vi "New From Listener.vi"(4 "Immutable TLS":refnum<k36>, 6 "TLS":bool, 7 "From":refnum<class "Endpoint.lvclass">, 10 "TCP Connection":refnum<k5>, 11 "URI":refnum<class "URI.lvclass">) -> (0 "error out":errorcluster, 3 "Client":refnum<class "Websocket Client.lvclass">)   [LabVIEW 2020, in "Stream-Websocket.lvlib" / "Websocket Client.lvclass"]
uses:
  Websocket Client.lvclass
  <vilib>/IlluminatedG/lv-stream/URI/URI.lvclass
  <vilib>/IlluminatedG/lv-stream/Endpoint/Endpoint.lvclass
  C:/Program Files (x86)/National Instruments/LabVIEW 2020/vi.lib/IlluminatedG/lv-stream/Endpoint/Endpoint.lvclass
  C:/Program Files (x86)/National Instruments/LabVIEW 2020/vi.lib/IlluminatedG/lv-stream/Connection/Connection.lvclass
  Websocket Client.lvclass/Websocket Client.ctl
  <vilib>/IlluminatedG/lv-stream/Connection State.ctl
  <vilib>/IlluminatedG/lv-stream/Connection/State.ctl
  <vilib>/IlluminatedG/lv-stream/Stream.lvlib
  <vilib>/IlluminatedG/lv-stream/Connection/Connection.lvclass
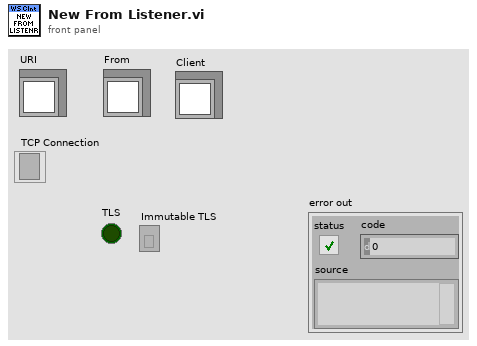
[diagram p1: front panel]
types:
  T1 = typedef "Stream.lvlib/Connection.lvclass/State.ctl" = enum16{"Closed", "Idle", "Connecting", "Connected", "Shutdown"}
  T2 = typedef "Stream.lvlib/Connection State.ctl" = enum16{"Connected", "Disconnected"}
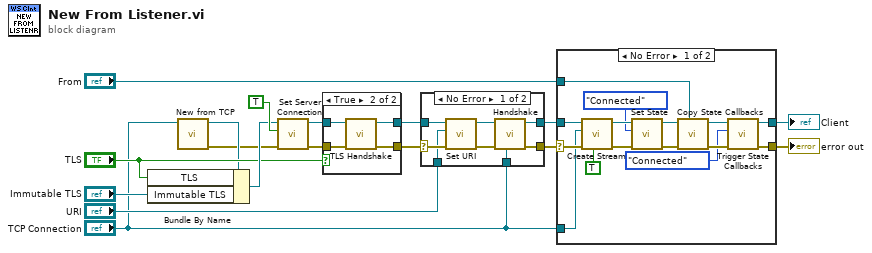
[diagram p0: block diagram]
diagram:
  n1 = call "New from TCP.vi"("TCP Connection"="TCP Connection") -> ("error out"=w2:errorcluster, "Websocket Client out"=w3:refnum<class "Websocket Client.lvclass">)  [unwired: 9 in]
  n2 = Bundle By Name(cluster=w3, "TLS"="TLS", "Immutable TLS"="Immutable TLS") -> (w9:refnum<class "Websocket Client.lvclass">)
  n3 = call "Set Server Connection.vi"("error in (no error)"=w2, "Server Connection"=TRUE, "Websocket Client in"=w9) -> ("error out"=w7:errorcluster, "Websocket Client out"=w8:refnum<class "Websocket Client.lvclass">)  [unwired: 7 in]
  n4 = case shown="True" "TLS" {
    tunnel: w8 -> [w18 w23]
    tunnel: w7 -> [w19 w22]
    tunnel: [w19 w21] -> w6
    tunnel: [w18 w20] -> w5
    frame False {
    }
    frame True {
      n5 = call "TLS Handshake.vi"("error in (no error)"=w22, "Websocket Client in"=w23) -> ("error out"=w21:errorcluster, "Websocket Client out"=w20:refnum<class "Websocket Client.lvclass">)  [unwired: 8 in]
    }
  }
  n6 = case shown="No Error" w6 {
    selector: w6 -> [w31 w33]
    tunnel: "URI" -> [w30 _]
    tunnel: [w27 w33] -> w13
    tunnel: [w26 w32] -> w12
    tunnel: "TCP Connection" -> [w25 _]
    tunnel: w5 -> [w24 w32]
    frame No Error {
      n7 = call <vilib>:"Set URI.vi"("error in (no error)"=w31, "URI"=w30, "Endpoint in"=w24) -> ("error out"=w28:errorcluster, "Endpoint out"=w29:refnum<class "Websocket Client.lvclass">)  [unwired: 7 in]
      n8 = call "Handshake.vi"("TCP Connection"=w25, "error in (no error)"=w28, "Websocket Client in"=w29) -> ("error out"=w27:errorcluster, "Websocket Client out"=w26:refnum<class "Websocket Client.lvclass">)  [unwired: 7 in]
    }
    frame Error {
    }
  }
  n9 = case shown="No Error" w13 {
    selector: w13 -> [w47 w49]
    tunnel: w12 -> [w48 w50]
    tunnel: "TCP Connection" -> [w46 _]
    tunnel: "From" -> [w38 _]
    tunnel: [w37 w50] -> w15
    tunnel: [w36 w49] -> w14
    frame No Error {
      n10 = call "Create Stream.vi"("Server Stream"=TRUE, "error in (no error)"=w47, "TCP Connection"=w46, "Websocket Client in"=w48) -> ("error out"=w39:errorcluster, "Websocket Client out"=w40:refnum<class "Websocket Client.lvclass">)  [unwired: 6 in]
      n11 = call <vilib>:"Set State.vi"("error in (no error)"=w39, "State"=State."Connected", "Connection in"=w40) -> ("error out"=w42:errorcluster, "Connection out"=w41:refnum<class "Websocket Client.lvclass">)  [unwired: 7 in]
      n12 = call <vilib>:"Copy State Callbacks.vi"("From"=w38, "error in (no error)"=w42, "Endpoint in"=w41) -> ("error out"=w44:errorcluster, "Endpoint out"=w45:refnum<class "Websocket Client.lvclass">)  [unwired: 7 in]
      n13 = call <vilib>:"Trigger State Callbacks.vi"("error in (no error)"=w44, "State"=Connection_State."Connected", "Connection in"=w45) -> ("error out"=w36:errorcluster, "Connection out"=w37:refnum<class "Websocket Client.lvclass">)  [unwired: 7 in]
    }
    frame Error {
    }
  }
  "Client" <- w15
  "error out" <- w14
